vi "FRCts20_Backend_INI_CompetitionFGV.vi"(10 "Set?":bool, 11 "Value in":string) -> (3 "Value out":string)   [LabVIEW 2014, in "FRCts20_Backend_Engine.lvlib" / "FRCts20_Backend_INI Controller.lvclass"]
uses:
  FRCts20_Backend_INI Controller.lvclass
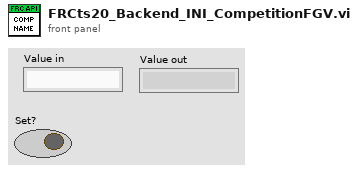
[diagram p1: front panel]
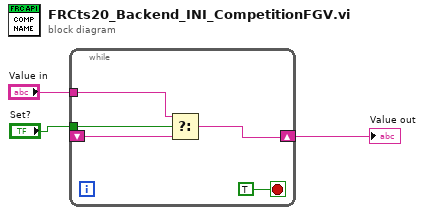
[diagram p0: block diagram]
diagram:
  n1 = while {
    tunnel: "Set?" -> [w8]
    tunnel: "Value in" -> [w7]
    shift-right: [w6] -> w3
    shift-left: _ -> [w5]
    stop <- TRUE stop-if-true
    n2 = Select(t=w7, s=w8, f=w5) -> (s? t:f=w6:string)
  }
  "Value out" <- w3
